vi "Tree Control - Traverse Configuration.vi"(7 "tree refnum":refnum<vi>, 8 "error in (no error)":errorcluster, 11 "virtual device":string) -> (0 "error out":errorcluster, 3 "virtual device out":string)   [LabVIEW 2023, in "SwitchExecController.lvlib"]
uses:
  SwitchExecController.lvlib
  <vilib>/SwitchExecutive/niseCfg.llb/niseCfg Get Virtual Device.vi
  <vilib>/SwitchExecutive/niseCfg.llb/niseVirtualDevice Get Route Groups.vi
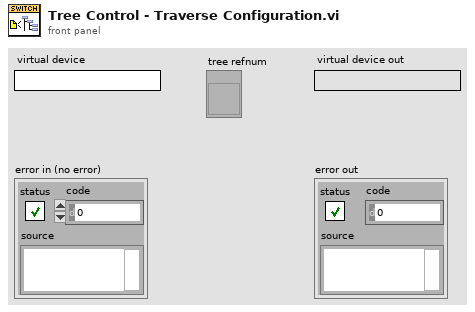
[diagram p1: front panel]
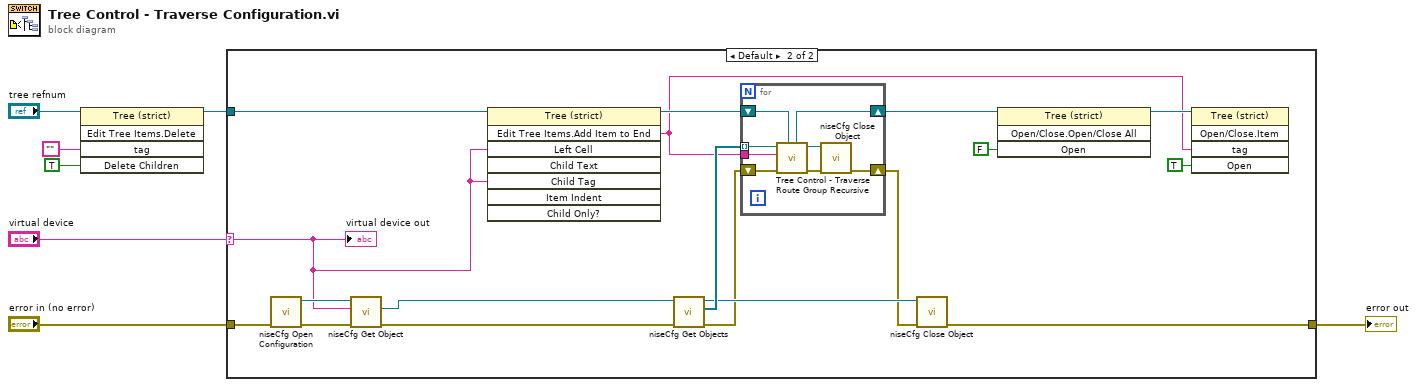
[diagram p0: block diagram]
diagram:
  n1 = invoke class="Tree (strict)" method="Edit Tree Items.Delete"(reference="tree refnum", "tag"="", "Delete Children"=TRUE ("Delete Children?")) -> (reference out=w5:refnum<vi>)  [unwired: 2 in, 4 out]
  n2 = case shown="Default" "virtual device" {
    selector: "virtual device" -> [_ w14]
    tunnel: w5 -> [_ w21]
    tunnel: [w8 w16] -> w4
    tunnel: "error in (no error)" -> [w8 w15]
    frame "" {
    }
    frame Default {
      n3 = call <vilib>:"niseCfg Open Configuration.vi"("error in (no error)"=w15) -> ("error out"=w22:errorcluster, "niseCfg"=w23:refnum<k7>)  [unwired: 9 in]
      n4 = call-poly <vilib>:"niseCfg Get Object.vi"("error in (no error)"=w22, "Virtual Device Name"=w14, "niseCfg"=w23) -> ("error out"=w25:errorcluster, "Virtual Device"=w24:refnum<k7>)  [unwired: 6 in, 1 out]
      n5 = invoke class="Tree (strict)" method="Edit Tree Items.Add Item to End"(reference=w21, "Left Cell"=w14, "Child Tag"=w14) -> (reference out=w20:refnum<vi>, "Edit Tree Items:Add Item to End"=w10:string)  [unwired: 5 in, 6 out]
      n6 = call-poly <vilib>:"niseCfg Get Objects.vi"("error in (no error)"=w25, "Virtual Device"=w24) -> ("error out"=w18:errorcluster, "Route Groups"=w26:refnum<k7>[], "Virtual Device out"=w19:refnum<k7>)  [unwired: 7 in]
      n7 = for {
        tunnel: w26 -> [w32] mode=indexing
        shift-right: [w33] -> w13
        shift-left: w20 -> [w34]
        tunnel: w10 -> [w31]
        shift-right: [w27] -> w17
        shift-left: w18 -> [w28]
        n8 = call "Tree Control - Traverse Route Group Recursive.vi"("tree refnum"=w34, "error in (no error)"=w28, "parent tag"=w31, "Route Group"=w32) -> ("error out"=w29:errorcluster, "Route Group out"=w30:refnum<k7>, "tree refnum out"=w33:refnum<vi>)  [unwired: 5 in]
        n9 = call <vilib>:"niseCfg Close Object.vi"("error in (no error)"=w29, "Reference"=w30) -> ("error out"=w27:errorcluster)  [unwired: 9 in]
      }
      n10 = call <vilib>:"niseCfg Close Object.vi"("error in (no error)"=w17, "Reference"=w19) -> ("error out"=w16:errorcluster)  [unwired: 9 in]
      n11 = invoke class="Tree (strict)" method="Open/Close.Open/Close All"(reference=w13, "Open"=FALSE ("Open?")) -> (reference out=w11:refnum<vi>)  [unwired: 2 in, 3 out]
      n12 = invoke class="Tree (strict)" method="Open/Close.Item"(reference=w11, "tag"=w10, "Open"=TRUE ("Open?")) -> ()  [unwired: 2 in, 5 out]
      "virtual device out" <- w14
    }
  }
  "error out" <- w4
